vi "Autonomous A1 Center-EitherSwitch.vi"   [LabVIEW 2017]
uses:
  Framework/Robot Global Data.vi
types:
  T1 = typedef "Command Status Info.ctl" = cluster{"Name":string, "Status":T2, "notifier out":T3}
  T2 = typedef "Completion Status.ctl" = enum16{"Successful", "Aborted", "Incomplete"}
  T3 = typedef "Completion Notifier.ctl" = refnum<notifier>
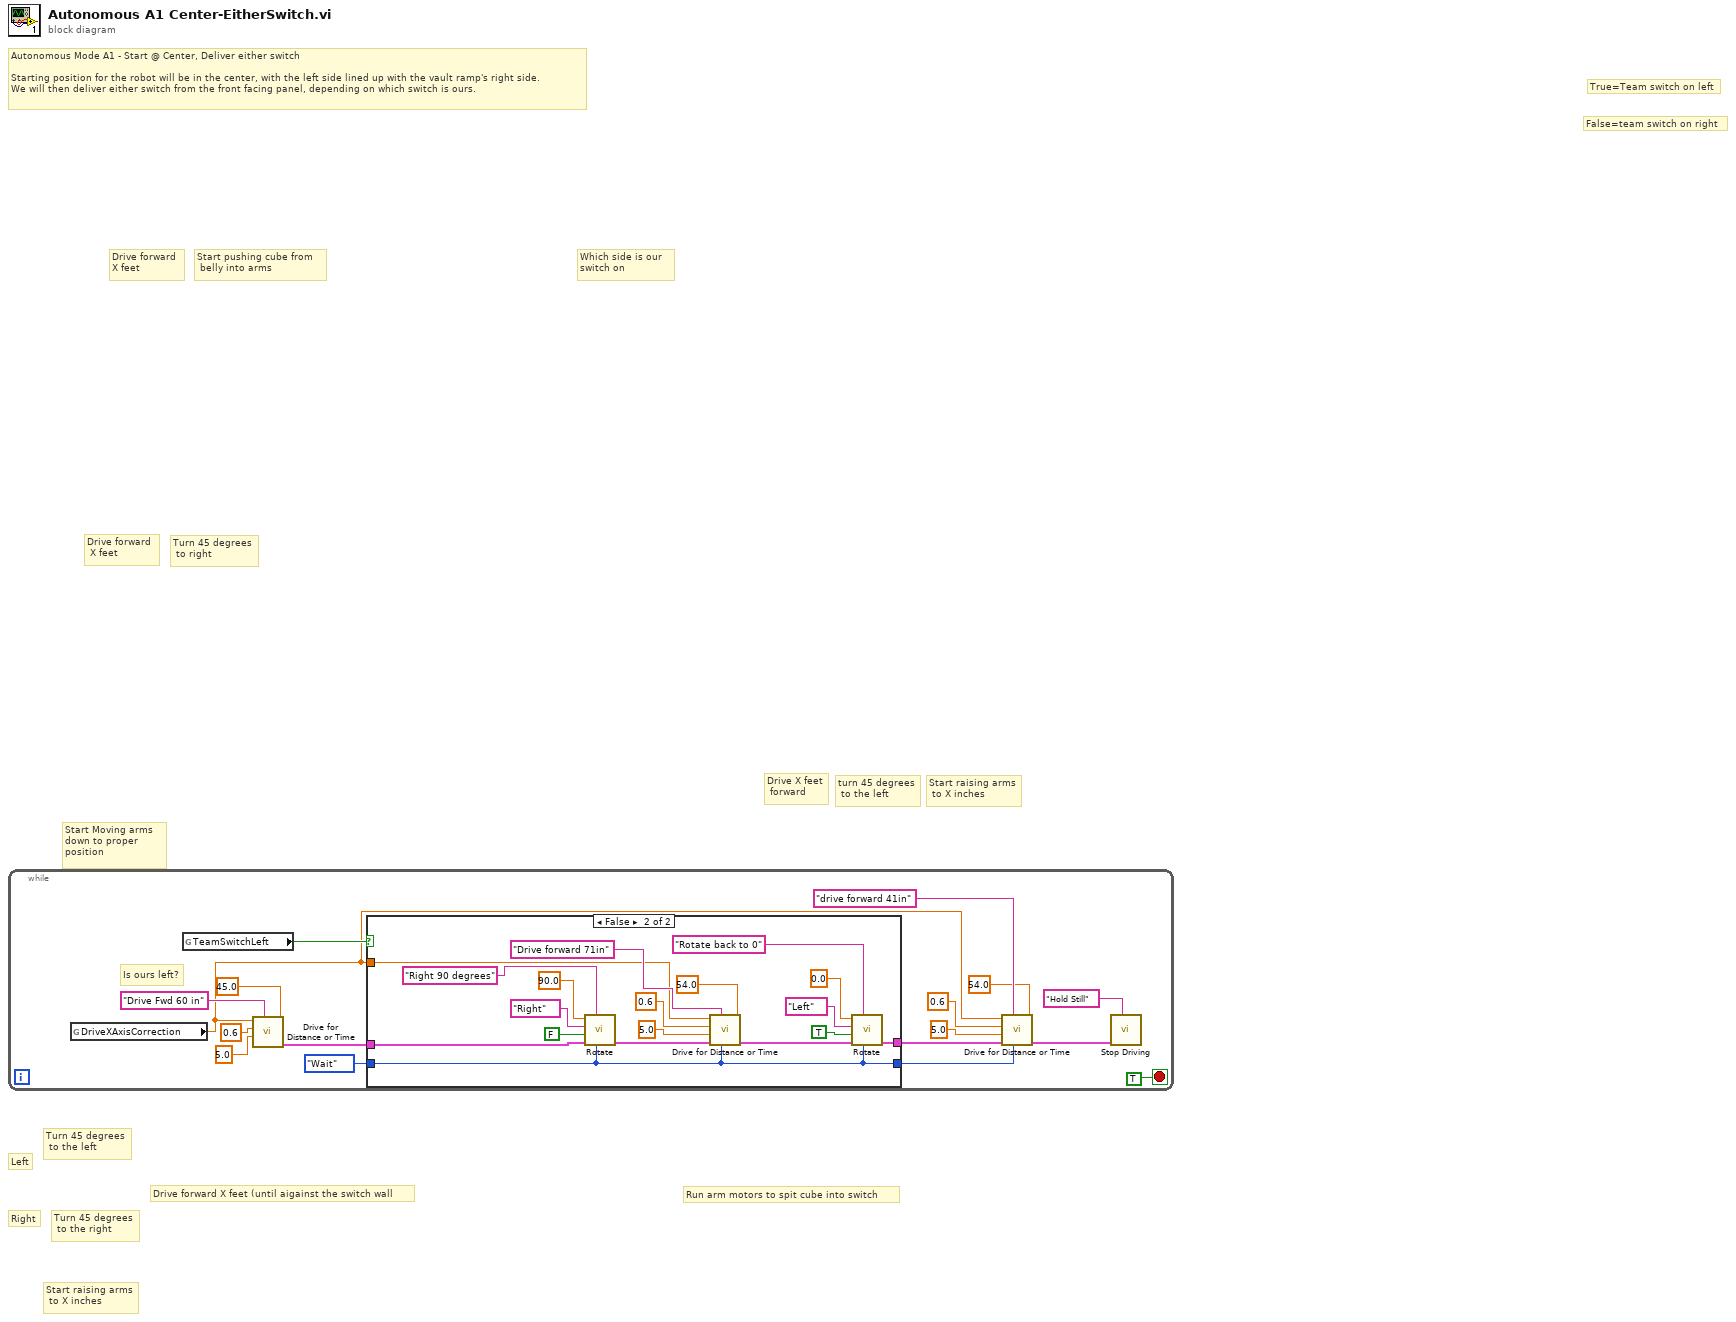
[diagram p0: block diagram]
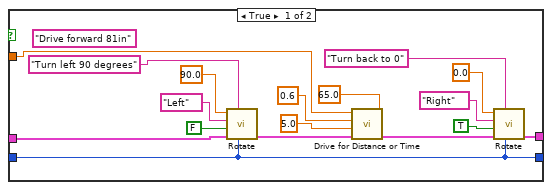
[diagram p2: hidden frame]
diagram:
  # "False=team switch on right"
  # "True=Team switch on left"
  # "Run arm motors to spit cube into switch"
  # "Drive forward X feet (until aigainst the switch wall"
  # "Start raising arms\n to X inches"
  # "turn 45 degrees\n to the left"
  # "Drive X feet\n forward"
  # "Turn 45 degrees\n to the right"
  # "Right"
  # "Start raising arms\n to X inches"
  # "Turn 45 degrees\n to right"
  # "Drive forward\n X feet"
  # "Turn 45 degrees\n to the left"
  # "Left"
  # "Which side is our \nswitch on"
  # "Start pushing cube from\n belly into arms"
  # "Drive forward\nX feet"
  # "Autonomous Mode A1 - Start @ Center, Deliver either switch\n\nStarting position for the robot will be in the center, with the left side lined up with the vault ramp's right side. \nWe will then deliver either switch from the front facing panel, depending on which switch is ours."
  # "Start Moving arms \ndown to proper \nposition"
  n1 = while {
    stop <- TRUE stop-if-true
    # "Is ours left?"
    n2 = global read "Robot Global Data.vi" "DriveXAxisCorrection"() -> (w1:dbl)
    n3 = global read "Robot Global Data.vi" "TeamSwitchLeft"() -> (w13:bool)
    n4 = call "Drive for Distance or Time.vi"("Distance (inches)"=45.0, "Description"="Drive Fwd 60 in", "Seconds"=5.0 ("Delay (s)"), "Y-axis"=0.6 ("Right Speed"), "X-axis"=w1) -> ("Command Info Out"=w6:T1)  [unwired: 6 in]
    n5 = case shown="False" w13 {
      tunnel: [w31 w49] -> w9
      tunnel: enum16{"Start", "Wait"}."Wait" ("Synchronication") -> [w30 w44]
      tunnel: [w30 w44] -> w12
      tunnel: w6 -> [w26 w41]
      tunnel: w1 -> [w18 w35]
      frame True {
        (unwired) "Drive forward 81in" ("Description")
        n6 = call "Rotate.vi"("Synchronication"=w30, "Description"="Turn left 90 degrees", "Command Info In"=w26, "Force Degrees"=FALSE, "Turn Direction"="Left" ("Direction"), "Degrees"=90.0) -> ("Command Info Out"=w23:T1)  [unwired: 5 in]
        n7 = call "Drive for Distance or Time.vi"("Distance (inches)"=65.0, "Command Info In"=w23, "Seconds"=5.0, "Y-axis"=0.6 ("Right Speed"), "X-axis"=w18) -> ("Command Info Out"=w19:T1)  [unwired: 6 in]
        n8 = call "Rotate.vi"("Synchronication"=w30, "Description"="Turn back to 0", "Command Info In"=w19, "Force Degrees"=TRUE, "Turn Direction"="Right" ("Direction"), "Degrees"=0.0) -> ("Command Info Out"=w31:T1)  [unwired: 5 in]
      }
      frame False {
        n9 = call "Rotate.vi"("Synchronication"=w44, "Description"="Right 90 degrees", "Command Info In"=w41, "Force Degrees"=FALSE, "Turn Direction"="Right" ("Direction"), "Degrees"=90.0) -> ("Command Info Out"=w42:T1)  [unwired: 5 in]
        n10 = call "Drive for Distance or Time.vi"("Distance (inches)"=54.0, "Synchronication"=w44, "Description"="Drive forward 71in", "Command Info In"=w42, "Seconds"=5.0, "Y-axis"=0.6 ("Seconds"), "X-axis"=w35) -> ("Command Info Out"=w43:T1)  [unwired: 4 in]
        n11 = call "Rotate.vi"("Synchronication"=w44, "Description"="Rotate back to 0", "Command Info In"=w43, "Force Degrees"=TRUE, "Turn Direction"="Left" ("Direction"), "Degrees"=0.0) -> ("Command Info Out"=w49:T1)  [unwired: 5 in]
      }
    }
    n12 = call "Drive for Distance or Time.vi"("Distance (inches)"=54.0, "Synchronication"=w12, "Description"="drive forward 41in", "Command Info In"=w9, "Seconds"=5.0, "Y-axis"=0.6 ("Right Speed"), "X-axis"=w1) -> ("Command Info Out"=w14:T1)  [unwired: 4 in]
    n13 = call "Stop Driving.vi"("Description"="Hold Still", "Command Info In"=w14) -> ()  [unwired: 9 in, 1 out]
  }
